vi "MouseclickAutoPhase.vi"(10 "error in (no error)":errorcluster) -> (2 "error out":errorcluster)   [LabVIEW 2014]
panel:
  in  "AutoItX3Lib.IAutoItX3":refnum<k7>
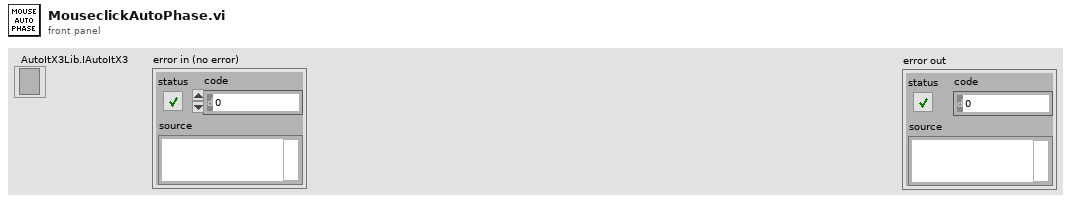
[diagram p1: front panel]
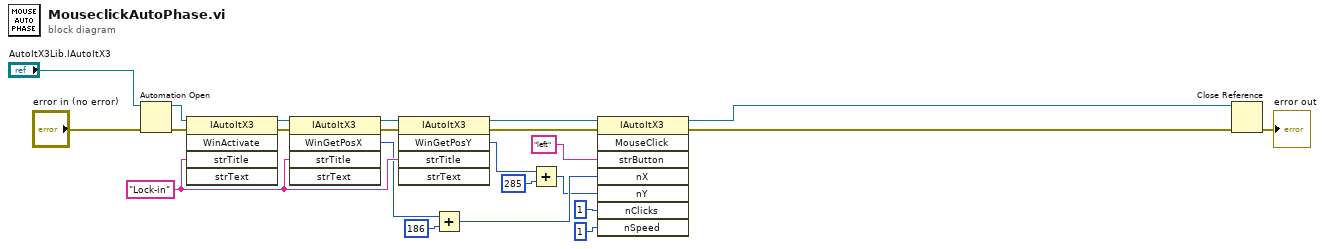
[diagram p0: block diagram]
diagram:
  w15 = "Lock-in" ("strTitle")
  n1 = Automation Open(error in (no error)="error in (no error)", Automation Refnum="AutoItX3Lib.IAutoItX3") -> (Automation Refnum=w21:refnum<k7>, error out=w20:errorcluster)  [unwired: 2 in]
  n2 = invoke class="IAutoItX3" method="WinActivate"(reference=w21, error in=w20, "strTitle"=w15) -> (reference out=w19:refnum<k7>, error out=w18:errorcluster)  [unwired: 2 in, 3 out]
  n3 = invoke class="IAutoItX3" method="WinGetPosX"(reference=w19, error in=w18, "strTitle"=w15) -> (reference out=w17:refnum<k7>, error out=w16:errorcluster, "WinGetPosX"=w13:i32)  [unwired: 2 in, 2 out]
  n4 = invoke class="IAutoItX3" method="WinGetPosY"(reference=w17, error in=w16, "strTitle"=w15) -> (reference out=w7:refnum<k7>, error out=w6:errorcluster, "WinGetPosY"=w14:i32)  [unwired: 2 in, 2 out]
  n5 = Add(x=w13, y=186) -> (x+y=w9:i32)
  n6 = Add(x=w14, y=285) -> (x+y=w8:i32)
  n7 = invoke class="IAutoItX3" method="MouseClick"(reference=w7, error in=w6, "strButton"="left", "nX"=w9, "nY"=w8, "nClicks"=1, "nSpeed"=1) -> (reference out=w1:refnum<k7>, error out=w2:errorcluster)  [unwired: 1 in, 6 out]
  n8 = Close Reference(reference=w1, error in (no error)=w2) -> (error out=→"error out":errorcluster)
